vi "AlliGator Get Decay Fit Parameter Map Data.vi"(6 "Map index":i32, 7 "Compute Decay Fit Parameter Map":bool, 8 "Error In":errorcluster, 9 "Y Resolution":i32, 10 "X Resolution":i32, 11 "Multiple Decays Fit Parameters":dbl[][](array[numeric])) -> (0 "Error Out":errorcluster, 2 "New Map Selected?":bool, 3 "Map Data (V x H)":dbl[][](array[numeric]))   [LabVIEW 2021, in "AlliGator Decay Fit Parameter Map.lvlib"]
doc: "Fills in matrix with fit parameter wherever it has been computed, NaN otherwise."
uses:
  AlliGator Decay Fit Parameter Map.lvlib
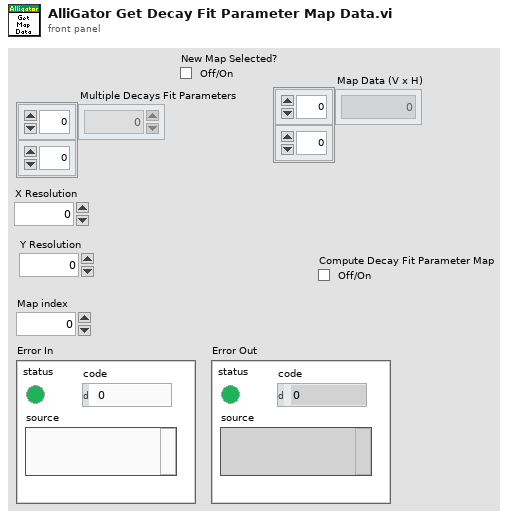
[diagram p1: front panel]
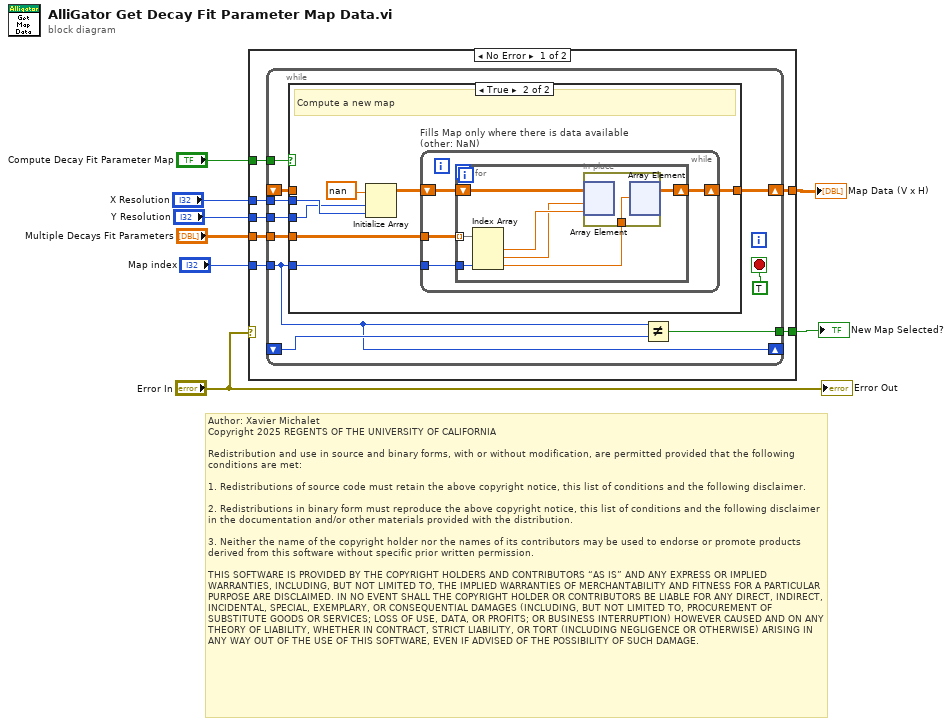
[diagram p0: block diagram]
diagram:
  # "Author: Xavier Michalet\nCopyright 2025 REGENTS OF THE UNIVERSITY OF CALIFORNIA\n\nRedistribution and use in source and binary forms, with or without modification, are permitted provided that the following conditions are met:\n\n1. Redistributions of source code must retain the above copyright notice, this list of conditions and the following disclaimer.\n\n2. Redistributions in binary form must reproduce the above copyright notice, this list of conditions and the following disclaimer in the documentation and/or other materials provided with the distribution.\n\n3. Neither the name of the copyright holder nor the names of its contributors may be used to endorse or promote products derived from this software without specific prior written permission.\n\nTHIS SOFTWARE IS PROVIDED BY THE COPYRIGHT HOLDERS AND CONTRIBUTORS “AS IS” AND ANY EXPRESS OR IMPLIED WARRANTIES, INCLUDING, BUT NOT LIMITED TO, THE IMPLIED WARRANTIES OF MERCHANTABILITY AND FITNESS FOR A PARTICULAR PURPOSE ARE DISCLAIMED. IN NO EVENT SHALL THE COPYRIGHT HOLDER OR CONTRIBUTORS BE LIABLE FOR ANY DIRECT, INDIRECT, INCIDENTAL, SPECIAL, EXEMPLARY, OR CONSEQUENTIAL DAMAGES (INCLUDING, BUT NOT LIMITED TO, PROCUREMENT OF SUBSTITUTE GOODS OR SERVICES; LOSS OF USE, DATA, OR PROFITS; OR BUSINESS INTERRUPTION) HOWEVER CAUSED AND ON ANY THEORY OF LIABILITY, WHETHER IN CONTRACT, STRICT LIABILITY, OR TORT (INCLUDING NEGLIGENCE OR OTHERWISE) ARISING IN ANY WAY OUT OF THE USE OF THIS SOFTWARE, EVEN IF ADVISED OF THE POSSIBILITY OF SUCH DAMAGE."
  n1 = case shown="No Error" "Error In" {
    tunnel: "Y Resolution" -> [w15 _]
    tunnel: "X Resolution" -> [w14 _]
    tunnel: "Map index" -> [w13 _]
    tunnel: [w12 _] -> w5
    tunnel: [w11 _] -> w4
    tunnel: "Compute Decay Fit Parameter Map" -> [w10 _]
    tunnel: "Multiple Decays Fit Parameters" -> [w9 _]
    frame No Error {
      n2 = while {
        tunnel: w9 -> [w24]
        tunnel: w10 -> [w23]
        shift-right: [w25] -> w11
        shift-left: _ -> [w21]
        tunnel: w13 -> [w16]
        shift-right: [w16] -> _
        shift-left: _ -> [w20]
        tunnel: [w19] -> w12
        tunnel: w14 -> [w18]
        tunnel: w15 -> [w17]
        stop <- TRUE stop-if-true
        n3 = case shown="True" w23 {
          tunnel: [w26 w33] -> w25
          tunnel: w24 -> [_ w31]
          tunnel: w21 -> [w26 _]
          tunnel: w16 -> [_ w29]
          tunnel: w18 -> [_ w28]
          tunnel: w17 -> [_ w27]
          frame False {
            # "use old map"
          }
          frame True {
            # "Compute a new map"
            n4 = Initialize Array(nan, w27, w28) -> (w30:dbl[][])
            n5 = while "Fills Map only where there is data available (other: NaN)" {
              shift-right: [w38] -> w33
              shift-left: w30 -> [w35]
              tunnel: w31 -> [w36]
              tunnel: w29 -> [w34]
              stop <- TRUE stop-if-true
              n6 = for {
                shift-right: [w44] -> w38
                shift-left: w35 -> [w45]
                tunnel: w36 -> [w43] mode=indexing
                tunnel: w34 -> [w42]
                n7 = Index Array(array=w43, index #3=w42) -> (element #1=w40:dbl, element #2=w39:dbl, element #3=w41:dbl)  [unwired: 2 in]
                n8 = in-place {
                  in-place-border: w41 -> [w46]
                  n9 = in-place-array #1(w45, w39, w40) -> ()  [unwired: 1 out]
                  n10 = in-place-array #1(w46) -> (w44:dbl[][])  [unwired: 2 out]
                }
              }
            }
          }
        }
        n11 = Not Equal?(x=w16, y=w20) -> (x != y?=w19:bool)
      }
    }
    frame Error {
    }
  }
  "New Map Selected?" <- w5
  "Map Data (V x H)" <- w4
  "Error Out" <- "Error In"
